vi "Trim Both Whitespace.vi"(0 "string":string) -> (2 "trimmed string":string)   [LabVIEW 2020, in "Communicable State Machine.lvlib"]
doc: "Removes all ASCII white space (spaces, tabs, carriage returns, and linefeeds) from the beginning, end, or both ends of <B>string</B>. The Trim Whitespace VI does not remove double byte characters.\n\n<b>Inputs:</b>\n - <b>string</b>\n\n<b>Outputs:</b>\n - <b>trimmed string</b>"
uses:
  Communicable State Machine.lvlib
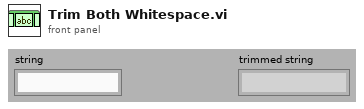
[diagram p1: front panel]
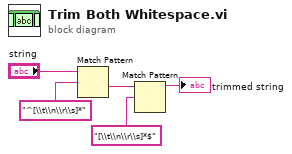
[diagram p0: block diagram]
diagram:
  n1 = Match Pattern(string="string", regular expression="^[\\t\\n\\r\\s]*") -> (after substring=w3:string)  [unwired: 1 in, 3 out]
  n2 = Match Pattern(string=w3, regular expression="[\\t\\n\\r\\s]*$") -> (before substring=→"trimmed string":string)  [unwired: 1 in, 3 out]
